vi "CgStart.vi"(3 "error in (no error)":errorcluster, 5 "VISA resource name":refnum<visa-resource-name>) -> (0 "error out":errorcluster, 2 "VISA resource name out":refnum<visa-resource-name>)   [LabVIEW 2009]
doc: "Starts streaming output from the cyberglove.\n\nSends an 'S' command to begin streaming data. Also, turns cyberglove light on."
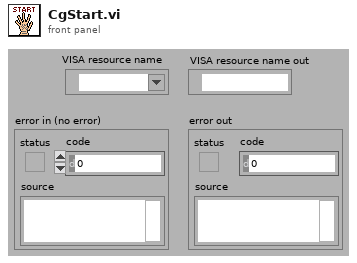
[diagram p1: front panel]
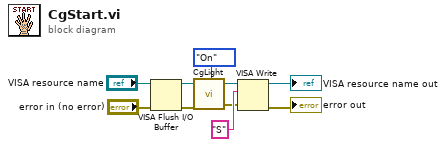
[diagram p0: block diagram]
diagram:
  n1 = VISA Flush I/O Buffer(VISA resource name="VISA resource name", error in (no error)="error in (no error)") -> (VISA resource name out=w6:refnum<visa-resource-name>, error out=w5:errorcluster)  [unwired: 1 in]
  n2 = call "CgLight.vi"("error in (no error)"=w5, "Mode"=enum16{"Off", "On", "Flash"}."On", "VISA resource name"=w6) -> ("error out"=w3:errorcluster, "VISA resource name out"=w4:refnum<visa-resource-name>)  [unwired: 2 in]
  n3 = VISA Write(VISA resource name=w4, write buffer="S", error in (no error)=w3) -> (VISA resource name out=→"VISA resource name out":refnum<visa-resource-name>, error out=→"error out":errorcluster)  [unwired: 1 out]
